vi "Wol_konfig new_to_old.vi"(11 "New Konfig in":T1) -> (3 "Old Konfig out":T4 {"Wolna Wykr num" items=["Brak", "Wykres 1", "Wykres 2", "Wykres 3", "Wykres 4"]})   [LabVIEW 2014]
uses:
  Kontrolki/GUI/RejWol_konfig.ctl
  Kontrolki/GUI/RejWol_typ.ctl
  Kontrolki/GUI/Wolna_WykrNum.ctl
  Kontrolki/GUI/RejWol_konfig_opis GUI.ctl
  Kontrolki/GUI/RejWol_numer_kanalu.ctl
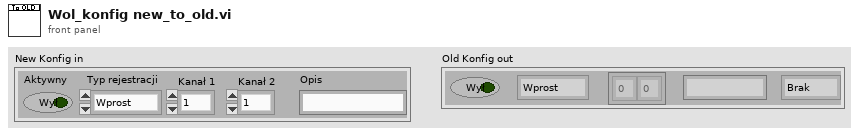
[diagram p1: front panel]
types:
  T1 = typedef "RejWol_konfig_opis GUI.ctl" = cluster{"Typ rejestracji":T2, "Opis":string, "Aktywny":bool, "Kanał 1":T3, "Kanał 2":T3}
  T2 = typedef "RejWol_typ.ctl" = enum16{"Wprost", "Moduł", "Kwadrat", "Iloczyn", "Faza"}
  T3 = typedef "RejWol_numer_kanalu.ctl" = enum16{"1", "2", "3", "4", "5", "6", "7", "8"}
  T4 = typedef "RejWol_konfig.ctl" = cluster{"Typ rejestracji":T2, "Kanały":i32[], "Opis":string, "Aktywny":bool, "Wolna Wykr num":T5}
  T5 = typedef "Wolna_WykrNum.ctl" = u16
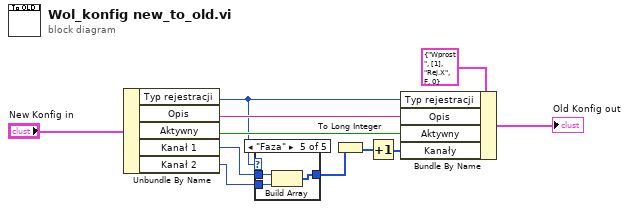
[diagram p0: block diagram]
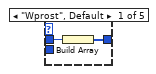
[diagram p2: hidden frame]
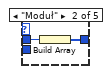
[diagram p3: hidden frame]
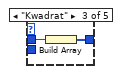
[diagram p4: hidden frame]
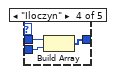
[diagram p5: hidden frame]
diagram:
  n1 = Unbundle By Name("New Konfig in") -> ("Typ rejestracji"=w2:T2, "Opis"=w9:string, "Aktywny"=w10:bool, "Kanał 1"=w6:T3, "Kanał 2"=w1:T3)
  n2 = case shown="\"Faza\"" w2 {
    tunnel: w6 -> [w13 w15 w17 w20 w23]
    tunnel: [w12 w14 w16 w19 w21] -> w5
    tunnel: w1 -> [_ _ _ w18 w22]
    frame "Wprost", Default {
      n3 = Build Array(w13) -> (w12:T3[])
    }
    frame "Moduł" {
      n4 = Build Array(w15) -> (w14:T3[])
    }
    frame "Kwadrat" {
      n5 = Build Array(w17) -> (w16:T3[])
    }
    frame "Iloczyn" {
      n6 = Build Array(w20, w18) -> (w19:T3[])
    }
    frame "Faza" {
      n7 = Build Array(w23, w22) -> (w21:T3[])
    }
  }
  n8 = To Long Integer(number=w5) -> (32bit integer=w4:i32[])
  n9 = Increment(x=w4) -> (x+1=w3:i32[])
  n10 = Bundle By Name(cluster=T4 {"Typ rejestracji"=enum."Wprost", "Kanały"=[1], "Opis"="Rej.X", "Aktywny"=FALSE, "Wolna Wykr num"=0} ("Rej.8"), "Typ rejestracji"=w2, "Opis"=w9, "Aktywny"=w10, "Kanały"=w3) -> (→"Old Konfig out":T4)
